vi "CambiarPtoDecimalString.vi"(1 "result":string[][](array[string])) -> (0 "result out":string[][](array[string]))   [LabVIEW 2019, in "Prueba05.lvclass"]
doc: "Cambia el punto decimal de un string desde \"punto\" a \"coma\" y lo vuelve a string"
uses:
  Prueba05.lvclass
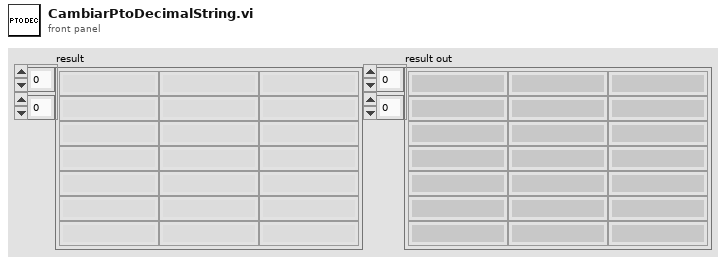
[diagram p1: front panel]
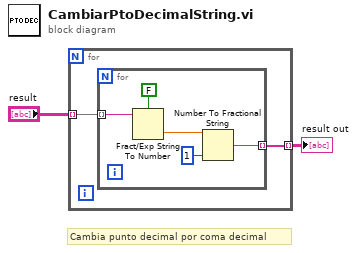
[diagram p0: block diagram]
diagram:
  # "Cambia punto decimal por coma decimal"
  n1 = for {
    tunnel: "result" -> [w4] mode=indexing
    tunnel: [w3] -> w1 mode=indexing
    n2 = for {
      tunnel: w4 -> [w9] mode=indexing
      tunnel: [w7] -> w3 mode=indexing
      n3 = Fract/Exp String To Number(use system decimal point (T)=FALSE, string=w9) -> (number=w8:dbl)  [unwired: 2 in, 1 out]
      n4 = Number To Fractional String(number=w8, precision (6)=i16 1) -> (F-format string=w7:string)  [unwired: 2 in]
    }
  }
  "result out" <- w1
